vi "Module Template Configuraton Extractor API.vi"(8 "error constant":errorcluster, 11 "App Cfg DVR":T2) -> (0 "error out":errorcluster, 3 "Module Template Config":T1)   [LabVIEW 2021, in "Controller.lvlib"]
doc: "This method extracts is a Poliphormic method used to read each module configuration."
uses:
  Controller.lvlib
  Architecture/Modules/Configuration/Typedefs/App Cfg DVR.ctl
  Architecture/Typedefs/Application Configuration.ctl
  Architecture/Modules/Module Template/Typedefs/Config.ctl
  Architecture/Modules/Core UI/Typedefs/Config.ctl
  Sound Manager/Typedefs/Config.ctl
  Typedefs/Config.ctl
  Architecture/Modules/Configuration/Configuration.lvlib
  Architecture/Modules/Core UI/Core UI.lvlib
  Sound Manager/Sound Manager.lvlib
  Architecture/Modules/Module Template/Module Template.lvlib
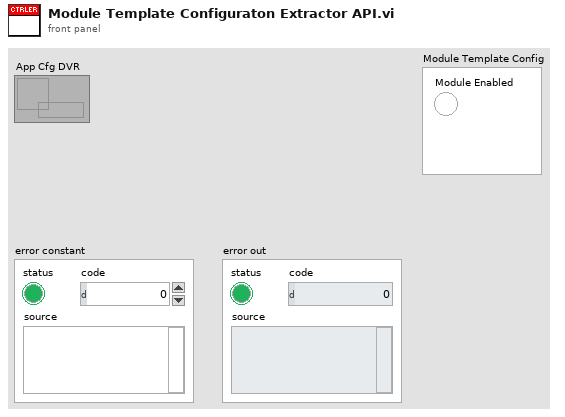
[diagram p1: front panel]
types:
  T1 = typedef "Controller.lvlib/Config.ctl" = cluster{"Module Enabled":bool}
  T2 = typedef "Configuration.lvlib/App Cfg DVR.ctl" = refnum<data-value>
  T3 = typedef "Configuration.lvlib/Application Configuration.ctl" = cluster{"Module Template Config":T4, "Core UI Config":T5, "Sound Manager Config":T6}
  T4 = typedef "Module Template.lvlib/Config.ctl" = cluster{"Module Enabled":bool}
  T5 = typedef "Core UI.lvlib/Config.ctl" = cluster{"Module Enabled":bool}
  T6 = typedef "Sound Manager.lvlib/Config.ctl" = cluster{"Sound Library Path":path, "dyn sounds path":path}
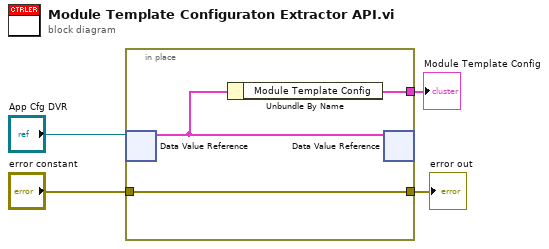
[diagram p0: block diagram]
diagram:
  n1 = in-place {
    in-place-border: [w5] -> w1
    in-place-border: "error constant" -> [w6]
    in-place-border: [w6] -> w2
    n2 = in-place-dvr #1("App Cfg DVR") -> (w7:T3)  [unwired: 1 out]
    n3 = Unbundle By Name(w7) -> ("Module Template Config"=w5:T4)
    n4 = in-place-dvr #1(w7) -> ()  [unwired: 2 out]
  }
  "error out" <- w2
  "Module Template Config" <- w1
